vi "Verify Terminals for Message Type.vi"(7 "message type":T3, 8 "error in":errorcluster, 10 "directions":string[](array[string]), 11 "terminals":T1[](array[typedef])) -> (0 "error out":errorcluster, 2 "Tx terminal":T1, 3 "Rx terminal":T1)   [LabVIEW 2020, in "MIL-STD 1553 Import.lvlib"]
uses:
  MIL-STD 1553 Import.lvlib
  Shared/Message Type.ctl
  Shared/Terminal Endpoint.ctl
  Shared/Address.ctl
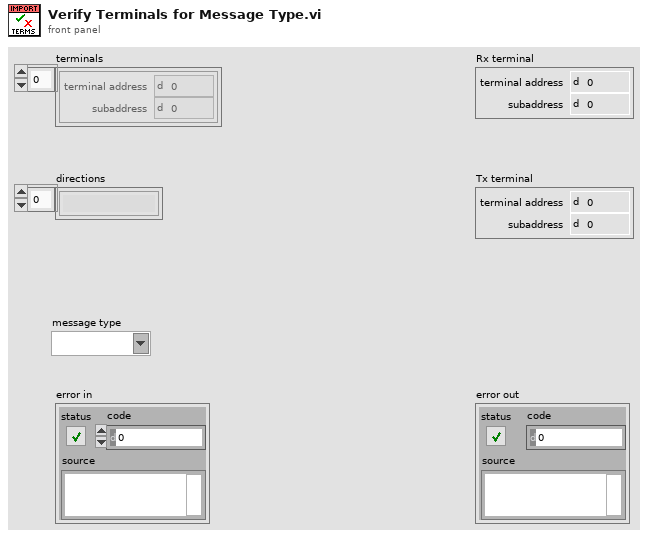
[diagram p1: front panel]
types:
  T1 = typedef "Terminal Endpoint.ctl" = cluster{"terminal address":T2, "subaddress":T2}
  T2 = typedef "Address.ctl" = u16
  T3 = typedef "Message Type.ctl" = string
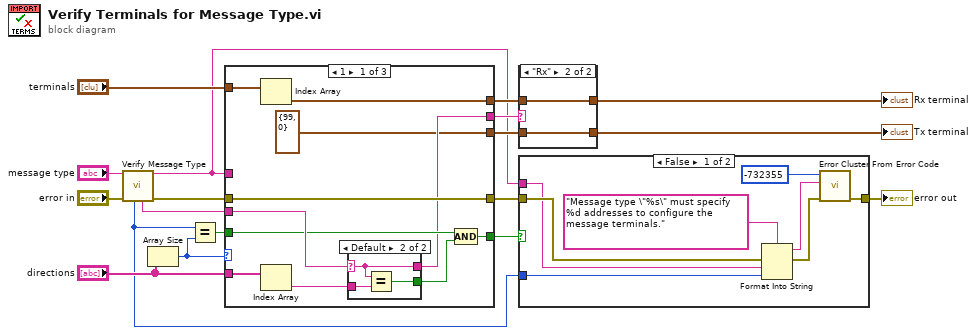
[diagram p0: block diagram]
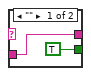
[diagram p2: hidden frame]
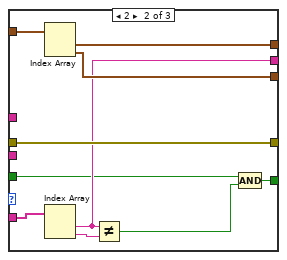
[diagram p3: hidden frame]
diagram:
  n1 = call "Verify Message Type.vi"("error in"="error in", "message type in"="message type") -> ("error out"=w8:errorcluster, "message type out"=w1:T3, "expected RT direction"=w10:string, "number of expected addresses"=w4:i32)  [unwired: 6 in]
  n2 = Array Size(array="directions") -> (size(s)=w7:i32)
  n3 = Equal?(x=w4, y=w7) -> (x = y?=w6:bool)
  n4 = case shown="1" w7 {
    tunnel: w8 -> [w26 w41 w45]
    tunnel: [w26 w41 w45] -> w2
    tunnel: "directions" -> [w29 w44 _]
    tunnel: "terminals" -> [w28 w43 _]
    tunnel: w10 -> [w25 _ _]
    tunnel: [w20 w40 _] -> w15
    tunnel: [T1 {"terminal address"=99, "subaddress"=0} ("terminal") w39 _] -> w16
    tunnel: [w21 w38 _] -> w14
    tunnel: w6 -> [w24 w37 _]
    tunnel: [w22 w35 _] -> w5
    tunnel: w1 -> [_ _ _]
    frame 1 {
      n5 = Index Array(array=w28) -> (element=w20:T1)  [unwired: 1 in]
      n6 = Index Array(array=w29) -> (element=w27:string)  [unwired: 1 in]
      n7 = case shown="Default" w25 {
        selector: w25 -> [_ w32]
        tunnel: w27 -> [w30 w34]
        tunnel: [TRUE w33] -> w23
        tunnel: [w30 w32] -> w21
        frame "" {
        }
        frame Default {
          n8 = Equal?(x=w32, y=w34) -> (x = y?=w33:bool)
        }
      }
      n9 = Compound Arithmetic op=AND(w24, w23) -> (w22:bool)
    }
    frame 2 {
      n10 = Index Array(array=w43) -> (element #1=w40:T1, element #2=w39:T1)  [unwired: 2 in]
      n11 = Index Array(array=w44) -> (element #1=w38:string, element #2=w42:string)  [unwired: 2 in]
      n12 = Not Equal?(x=w38, y=w42) -> (x != y?=w36:bool)
      n13 = Compound Arithmetic op=AND(w37, w36) -> (w35:bool)
    }
    frame Default {
    }
  }
  n14 = case shown="\"Rx\"" w14 {
    tunnel: w15 -> [w46 w49]
    tunnel: [w47 w49] -> w17
    tunnel: [w46 w48] -> w18
    tunnel: w16 -> [w47 w48]
    frame Default {
    }
    frame "Rx" {
    }
  }
  "Tx terminal" <- w18
  "Rx terminal" <- w17
  n15 = case shown="False" w5 {
    tunnel: w1 -> [w53 _]
    tunnel: w4 -> [w52 _]
    tunnel: [w50 w58] -> w3
    tunnel: w2 -> [w54 w58]
    frame False {
      n16 = Format Into String(format string="Message type \"%s\" must specify %d addresses to configure the message terminals.", error in=w54, w53, w52) -> (resulting string=w56:string, error out=w51:errorcluster)  [unwired: 1 in]
      n17 = call <vilib>:"Error Cluster From Error Code.vi"("error in (no error)"=w51, "error message (\"\")"=w56, "error code (0)"=-732355) -> ("error out"=w50:errorcluster)  [unwired: 6 in]
    }
    frame True {
    }
  }
  "error out" <- w3
